vi "test Deployment Import RT-Only Configuration.vi"(8 "error in":errorcluster, 11 "TestCase in":refnum<class "Deployment.lvclass">=refnum) -> (0 "error out":errorcluster, 3 "TestCase out":refnum<class "Deployment.lvclass">)   [LabVIEW 2020, in "Deployment.lvclass"]
uses:
  Deployment.lvclass
  <vilib>/addons/_JKI Toolkits/VI Tester/TestCase.llb/TestCase.lvclass
  315b1c3a-44c8-49e8-b756-01f865c29b4a.vi
  Scripting/AIM MIL-STD-1553 Scripting.lvlib
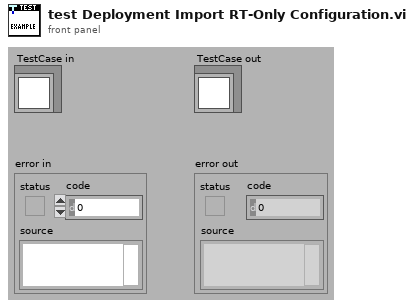
[diagram p1: front panel]
types:
  T1 = typedef "Custom Device API.lvlib/Custom Device Item Ref.ctl" = u64
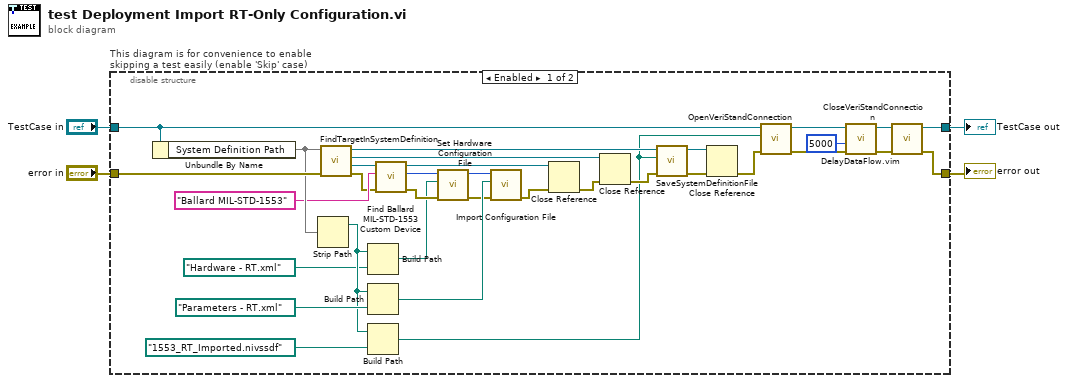
[diagram p0: block diagram]
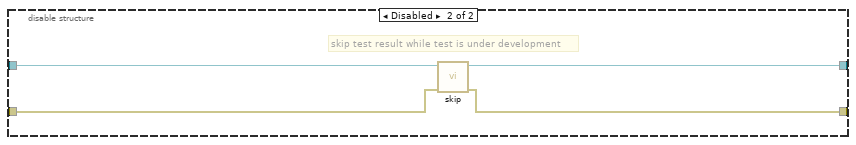
[diagram p2: hidden frame]
diagram:
  n1 = disable-structure "This diagram is for convenience to enable skipping a test easily (enable 'Skip' case)" shown="Enabled" {
    disable-tunnel: "TestCase in" -> [w30 w40]
    disable-tunnel: [w31 w38] -> w1
    disable-tunnel: [w33 w39] -> w3
    disable-tunnel: "error in" -> [w29 w37]
    frame Enabled {
      n2 = Unbundle By Name(w30) -> ("System Definition Path"=w27)
      n3 = Strip Path(path=w27) -> (stripped path=w11:path)  [unwired: 1 out]
      n4 = call "FindTargetInSystemDefinition.vi"("error in"=w29, "system definition path"=w27) -> ("error out"=w16:errorcluster, "Target"=w19:refnum<k24>, "Root"=w22:refnum<k24>, "System Definition"=w28:refnum<k24>)  [unwired: 6 in]
      n5 = Build Path(base path=w11, name or relative path=path "Hardware - RT.xml") -> (appended path=w5:path)
      n6 = Build Path(base path=w11, name or relative path=path "Parameters - RT.xml") -> (appended path=w12:path)
      n7 = Build Path(base path=w11, name or relative path=path "1553_RT_Imported.nivssdf") -> (appended path=w15:path)
      n8 = call "Find Ballard MIL-STD-1553 Custom Device.vi"("error in"=w16, "name"="Ballard MIL-STD-1553", "target in"=w19) -> ("error out"=w7:errorcluster, "Ballard MIL-STD 1553 custom device"=w9:T1, "target out"=w17:refnum<k24>)  [unwired: 5 in, 1 out]
      n9 = call "Set Hardware Configuration File.vi"("error in"=w7, "hardware configuration file path"=w5, "Ballard MIL-STD 1553 custom device in"=w9) -> ("error out"=w6:errorcluster, "Ballard MIL-STD 1553 custom device out"=w8:T1)  [unwired: 7 in]
      n10 = call "Import Configuration File.vi"("error in"=w6, "parameters configuration file path"=w12, "Ballard MIL-STD 1553 custom device in"=w8) -> ("error out"=w13:errorcluster)  [unwired: 7 in, 1 out]
      n11 = Close Reference(reference=w17, error in (no error)=w13) -> (error out=w20:errorcluster)
      n12 = Close Reference(reference=w22, error in (no error)=w20) -> (error out=w21:errorcluster)
      n13 = call "SaveSystemDefinitionFile.vi"("error in (no error)"=w21, "System Definition File in"=w15, "System Definition Reference in"=w28) -> ("error out"=w24:errorcluster, "System Definition Reference out"=w25:refnum<k24>)  [unwired: 7 in]
      n14 = Close Reference(reference=w25, error in (no error)=w24) -> (error out=w23:errorcluster)
      n15 = call-dynamic "OpenVeriStandConnection.vi"("error in (no error)"=w23, "System Definition File"=w15, "VeriStand Test Case in"=w30) -> ("error out"=w36:errorcluster, "VeriStand Test Case out"=w32:refnum<class "Deployment.lvclass">)  [unwired: 6 in, 1 out]
      n16 = call "DelayDataFlow.vim"("value in"=w36, "milliseconds to wait"=u32 5000) -> ("value out"=w34:errorcluster)  [unwired: 2 in, 1 out]
      n17 = call-dynamic "CloseVeriStandConnection.vi"("error in (no error)"=w34, "VeriStand Test Case in"=w32) -> ("error out"=w33:errorcluster, "VeriStand Test Case out"=w31:refnum<class "Deployment.lvclass">)  [unwired: 8 in]
    }
    frame Disabled {
      # "skip test result while test is under development"
      n18 = call <vilib>:"skip.vi"("error in (no error)"=w37, "TestCase in"=w40) -> ("error out"=w39:errorcluster, "TestCase out"=w38:refnum<class "TestCase.lvclass">)  [unwired: 8 in]
    }
  }
  "error out" <- w3
  "TestCase out" <- w1
